vi "PT3_Finish.vi"(4 "Input 1 Rate":i32, 6 "Input 0 Rate":i32, 7 "Stop Reason":enum16{"timeover", "manual", "overflow"}(ring), 8 "error in":errorcluster, 9 "Num Records":i32, 10 "Stop After (ms)":i32, 11 "refnum in":refnum<file>) -> (0 "error out":errorcluster)   [LabVIEW 8.6]
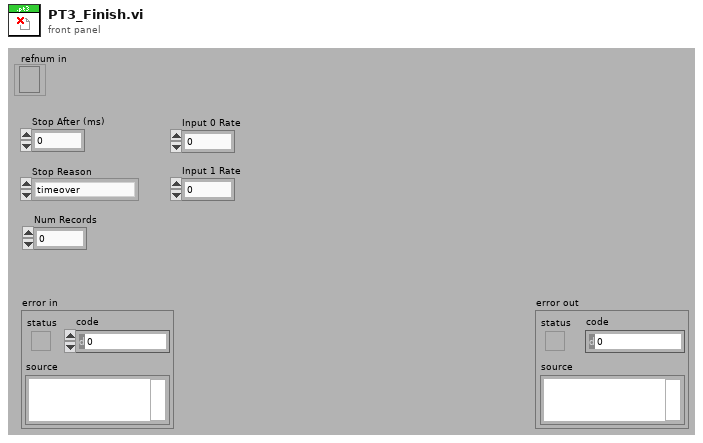
[diagram p1: front panel]
types:
  T1 = enum16{"big-endian, network order", "native, host order", "little-endian"}
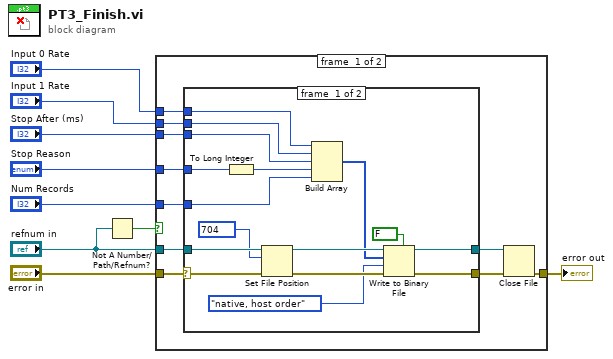
[diagram p0: block diagram]
diagram:
  n1 = Not A Number/Path/Refnum?(number/path/refnum="refnum in") -> (NaN/Path/Refnum?=w4:bool)
  n2 = case shown="False" w4 {
    tunnel: "error in" -> [w19 w38]
    tunnel: "refnum in" -> [w18 _]
    tunnel: [w17 w38] -> w8
    tunnel: "Stop Reason" -> [w14 _]
    tunnel: "Num Records" -> [w13 _]
    tunnel: "Stop After (ms)" -> [w12 _]
    tunnel: "Input 1 Rate" -> [w11 _]
    tunnel: "Input 0 Rate" -> [w10 _]
    frame #0 {
      n3 = case shown="No Error" w19 {
        selector: w19 -> [w35 w36]
        tunnel: w18 -> [w34 w37]
        tunnel: [w32 w36] -> w16
        tunnel: [w31 w37] -> w15
        tunnel: w14 -> [w28 _]
        tunnel: w13 -> [w25 _]
        tunnel: w12 -> [w27 _]
        tunnel: w11 -> [w21 _]
        tunnel: w10 -> [w20 _]
        frame #0 {
          n4 = To Long Integer(number=w28) -> (32bit integer=w26:i32)
          n5 = Set File Position(offset (in bytes) (0)=i64 704, refnum=w34, error in=w35) -> (refnum out=w30:refnum<file>, error out=w33:errorcluster)  [unwired: 1 out]
          n6 = Build Array(w20, w21, w27, w26, w25) -> (w24:i32[])
          n7 = Write to Binary File(file (use dialog)=w30, data=w24, error in=w33, 5:FALSE ("prepend array or string size? (T)"), 9:T1."native, host order" ("byte order (0:big-endian, network order)")) -> (refnum out=w31:refnum<file>, error out=w32:errorcluster)  [unwired: 2 out]
        }
        frame #1 {
        }
      }
      n8 = Close File(refnum=w15, error in=w16) -> (error out=w17:errorcluster)  [unwired: 1 out]
    }
    frame #1 {
    }
  }
  "error out" <- w8
